vi "Modify Desired Inverted (SubVI).vi"(9 "Nu des":dbl[](array[numeric])=[0.0, 0.0, 0.0, 0.0, 0.0, 0.0], 10 "Eta des":dbl[](array[numeric])=[0.0, 0.0, 0.5059668728304524, 0.0, 0.0, 0.0], 11 "r_off":dbl[](array[numeric])=[1.0, 1.0, 0.0]) -> (2 "nu_des_m":dbl[](array[numeric]), 3 "eta_des_m":dbl[](array[numeric]))   [LabVIEW 2014, in "Guidance Library.lvlib" / "Constant Jerk Guidance.lvclass"]
uses:
  Constant Jerk Guidance.lvclass
  <vilib>/imath/engines/lvmath2/RunTimeEngine/IndexRead/NIMS V(S).vi
  <instcachedir>/0/NIMS V(S)_0488751826AF41519A22953C041130DC.lvgen/NIMS V(S)_0488751826AF41519A22953C041130DC_000.vi
  <vilib>/imathl/engines/lvmath/Functions/Error Handling/Create Error.vi
  <vilib>/imath/engines/lvmath2/RunTimeEngine/IndexRead/NIMS V(R2).vi
  <instcachedir>/0/NIMS V(R2)_C76619605A0E4E9F8B2FA9389712AC47.lvgen/NIMS V(R2)_C76619605A0E4E9F8B2FA9389712AC47_000.vi
  <vilib>/imath/engines/lvmath2/RunTimeEngine/ArithmeticOperatorToken/NIMS_ArithmeticOperator_multmx(M,CV).vi
  <instcachedir>/0/NIMS_ArithmeticOperator_multmx(M,CV)_787B4652E60B4C52835A7FB23671E425.lvgen/NIMS_ArithmeticOperator_multmx(M,CV)_787B4652E60B4C52835A7FB23671E425_000.vi
  <vilib>/imath/engines/lvmath2/RunTimeEngine/ArithmeticOperatorToken/NIMS_ArithmeticOperator_plus.vi
  <instcachedir>/0/NIMS_ArithmeticOperator_plus_48D6EAACA5D645B09F7EC9C016C2DEA8.lvgen/NIMS_ArithmeticOperator_plus_48D6EAACA5D645B09F7EC9C016C2DEA8_003.vi
  <vilib>/imath/engines/lvmath2/RunTimeEngine/ErrorHandling/NIMS_Create Error From Enums.vi
  <vilib>/imath/engines/lvmath2/RunTimeEngine/MatrixToken/NIMS_MatrixToken_M_SorCV.vi
  <instcachedir>/0/NIMS_MatrixToken_M_SorCV_17569C4B859D4E2CA39B643FDD33E884.lvgen/NIMS_MatrixToken_M_SorCV_17569C4B859D4E2CA39B643FDD33E884_000.vi
  <vilib>/imath/engines/lvmath2/RunTimeEngine/NodeEndStatement/NIMS_NodeEndStatement_Output.vi
  <instcachedir>/0/NIMS_NodeEndStatement_Output_53EC0D466D134D7ABD903AC30B43404B.lvgen/NIMS_NodeEndStatement_Output_53EC0D466D134D7ABD903AC30B43404B_005.vi
  <vilib>/imath/engines/lvmath2/RunTimeEngine/ErrorHandling/NIMS_Finalize Error.vi
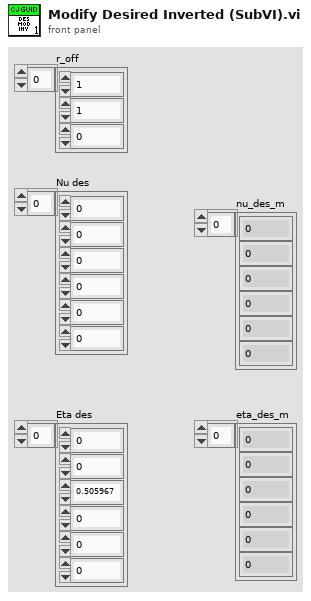
[diagram p1: front panel]
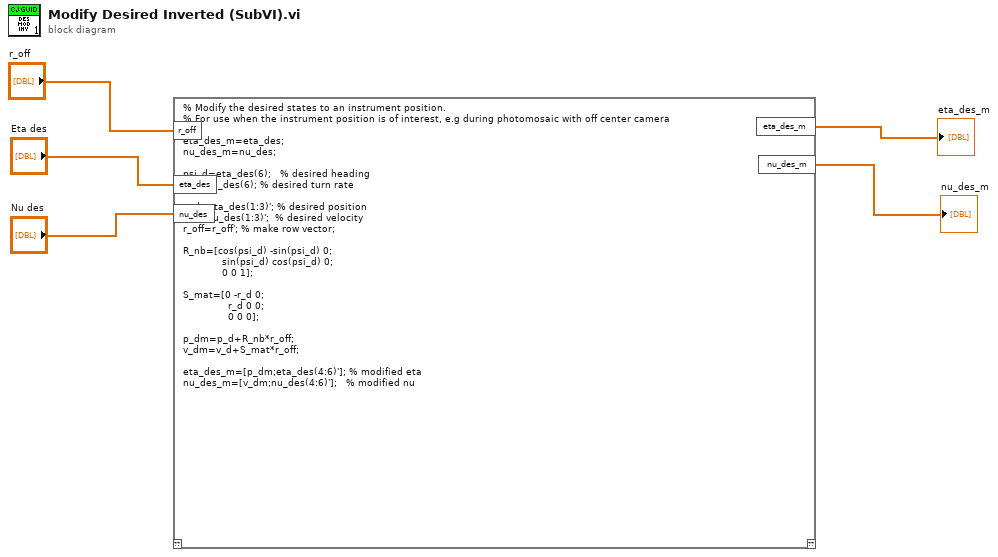
[diagram p0: block diagram]
diagram:
  n1 = mathscript code="% Modify the desired states to an instrument position. \n% For use when the instrument position is of interest, e.g during photomosaic with off center camera\n\neta_des_m=eta_des;\nnu_des_m=nu_des;\n\npsi_d=eta_des(6);   % desired heading\nr_d=nu_des(6); % desired turn rate\n\np_d=eta_des(1:3)'; % desired position\nv_d=nu_des(1:3)';  % desired velocity\nr_off=r_off'; % make row vector;\n\nR_nb=[cos(psi_d) -sin(psi_d) 0;\n             sin(psi_d) cos(psi_d) 0;\n             0 0 1];\n\nS_mat=[0 -r_d 0;\n               r_d 0 0;\n               0 0 0];\n\np_dm=p_d+R_nb*r_off;\nv_dm=v_d+S_mat*r_off;\n\neta_des_m=[p_dm;eta_des(4:6)']; % modified eta\nnu_des_m=[v_dm;nu_des(4:6)'];   % modified nu"("eta_des"="Eta des", "nu_des"="Nu des", "r_off"="r_off") -> ("eta_des_m"=→"eta_des_m":dbl[], "nu_des_m"=→"nu_des_m":dbl[])  [unwired: 1 in, 1 out]
